vi "Cesar.vi"() -> ()   [LabVIEW 2014]
uses:
  MyXControls/XControl 1.xctl
panel:
  in  "XControl 1":bool(xcontrol)
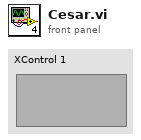
[diagram p1: front panel]
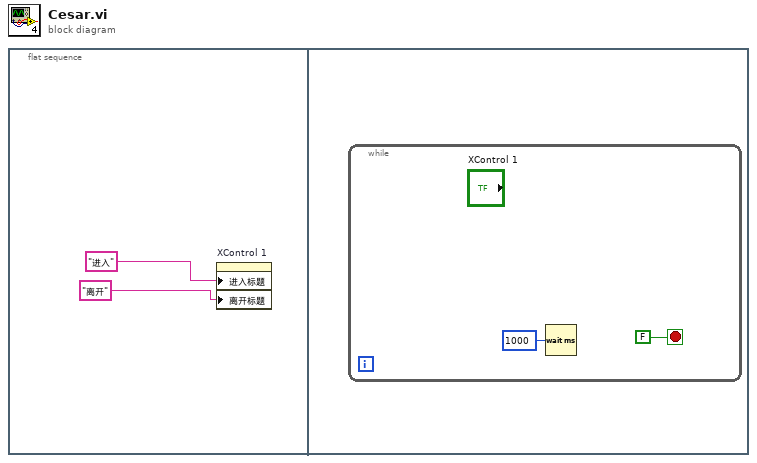
[diagram p0: block diagram]
diagram:
  n1 = flat-sequence {
    frame #0 {
      n2 = property on="XControl 1" class="XControl 1 (严格)"("进入标题"="进入", "离开标题"="离开") -> ()  [unwired: 2 in, 2 out]
    }
    frame #1 {
      n3 = while {
        stop <- FALSE stop-if-true
        n4 = Wait (ms)(milliseconds to wait=u32 1000 ("等待时间（毫秒）")) -> ()  [unwired: 1 out]
      }
    }
  }
